vi "Initialize Protection Frames.vi"(8 "error in (no error)":errorcluster, 10 "Frames":T1[](array[typedef]) {"Protection Configurations"."CRC Channels"."Data Type" items=["Signed", "Unsigned", "IEEE Float"]}, 11 "PCL (usec)":u32) -> (0 "error out":errorcluster, 2 "RT Frames":T8[](array[typedef]) {"Protection Configurations"."CRC Channels"."Data Type" items=["Signed", "Unsigned", "IEEE Float"]})   [LabVIEW 2015, in "Protection and Counter Support Engine.lvlib"]
uses:
  Protection and Counter Support Engine.lvlib
  Types/RT Frame Settings.ctl
  Shared/Types/Exported Frame Type.ctl
  Types/RT Protection Configuration.ctl
  Shared/Types/Protection Type.ctl
  Shared/Types/XNET Signal Configuration.ctl
  Shared/Types/Exported Counter Settings.ctl
  Shared/Types/Exported Event Trigger Type.ctl
  Shared/Types/Exported Frame Settings.ctl
  Shared/Types/Exported Protection Settings.ctl
  <vilib>/xnet/xnet.llb/XNET Create Session (Conversion).vi
  Shared/Protection and Counter Support Shared.lvlib
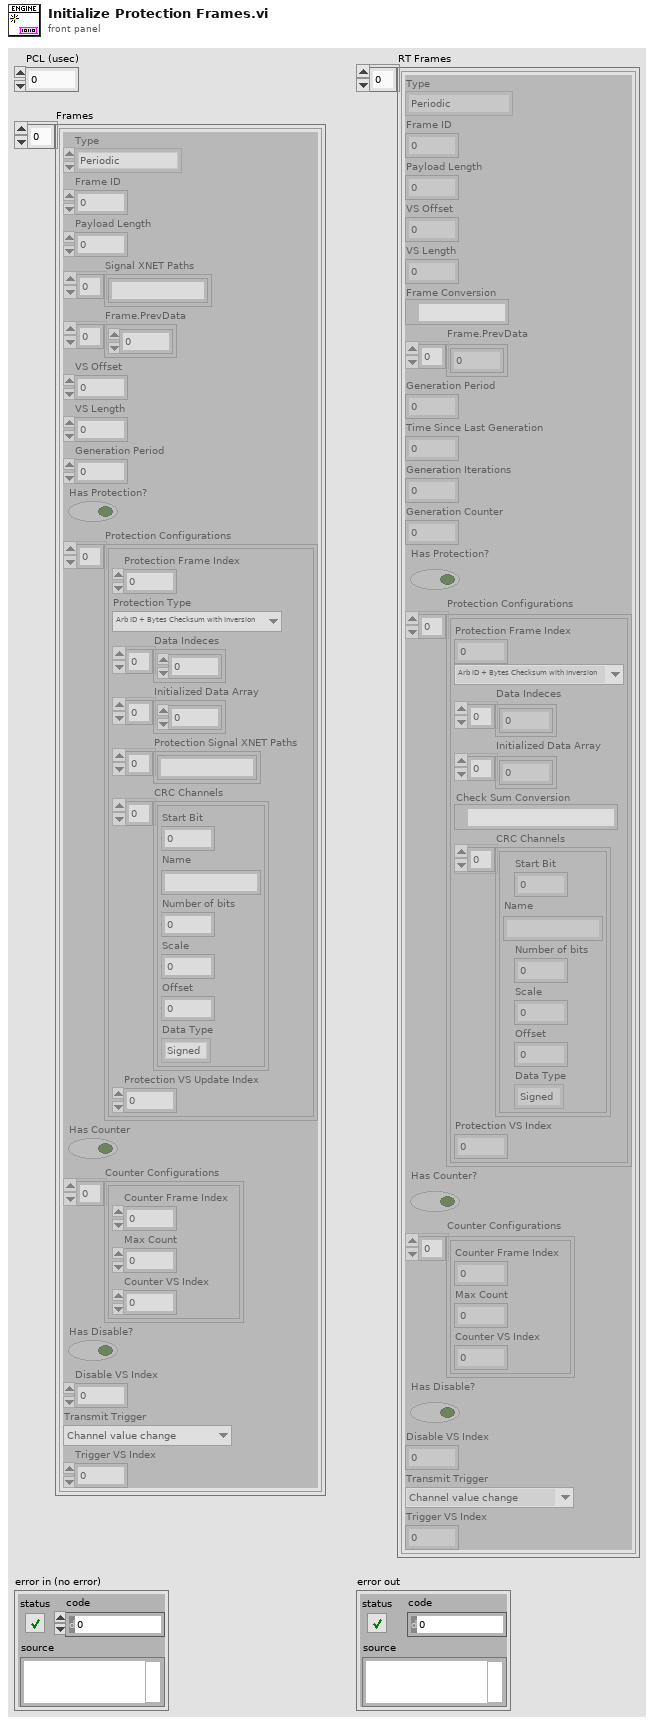
[diagram p1: front panel]
types:
  T1 = typedef "Protection and Counter Support Shared.lvlib/Exported Frame Settings.ctl" = cluster{"Type":T2, "Frame ID":u32, "Payload Length":u32, "Signal XNET Paths":string[], "Frame.PrevData":dbl[], "VS Offset":i32, "VS Length":i32, "Generation Period":u32, "Has Protection?":bool, "Protection Configurations":T3[], "Has Counter":bool, "Counter Configurations":T6[], "Has Disable?":bool, "Disable VS Index":i32, "Transmit Trigger":T7, "Trigger VS Index":i32}
  T2 = typedef "Protection and Counter Support Shared.lvlib/Exported Frame Type.ctl" = enum16{"Periodic", "Event", "Periodic/Event"}
  T3 = typedef "Protection and Counter Support Shared.lvlib/Exported Protection Settings.ctl" = cluster{"Protection Frame Index":i32, "Protection Type":T4, "Data Indeces":i32[], "Initialized Data Array":dbl[], "Protection Signal XNET Paths":string[], "CRC Channels":T5[], "Protection VS Update Index":i32}
  T4 = typedef "Protection and Counter Support Shared.lvlib/Protection Type.ctl" = enum16{"Arb ID + Bytes Checksum with Inversion", "Arb ID + Bytes CRC with Inversion", "Reversed Raw Signal Checksum with Inversion"}
  T5 = typedef "Protection and Counter Support Shared.lvlib/XNET Signal Configuration.ctl" = cluster{"Start Bit":i32, "Name":string, "Number of bits":i32, "Scale":dbl, "Offset":dbl, "Data Type":u32}
  T6 = typedef "Protection and Counter Support Shared.lvlib/Exported Counter Settings.ctl" = cluster{"Counter Frame Index":i32, "Max Count":dbl, "Counter VS Index":i32}
  T7 = typedef "Protection and Counter Support Shared.lvlib/Exported Event Trigger Type.ctl" = enum16{"Channel value change", "Trigger channel (not zero)", "Channel value change or trigger channel (not zero)", "Trigger channel (any value change)", "Channel value change or trigger channel (any value change)"}
  T8 = typedef "Protection and Counter Support Engine.lvlib/RT Frame Settings.ctl" = cluster{"Type":T2, "Frame ID":u32, "Payload Length":u32, "VS Offset":i32, "VS Length":i32, "Frame Conversion":refnum<k21>, "Frame.PrevData":dbl[], "Generation Period":u32, "Time Since Last Generation":u32, "Generation Iterations":u32, "Generation Counter":u32, "Has Protection?":bool, "Protection Configurations":T9[], "Has Counter?":bool, "Counter Configurations":T6[], "Has Disable?":bool, "Disable VS Index":i32, "Transmit Trigger":T7, "Trigger VS Index":i32}
  T9 = typedef "Protection and Counter Support Engine.lvlib/RT Protection Configuration.ctl" = cluster{"Protection Frame Index":i32, "Protection Type":T4, "Data Indeces":i32[], "Initialized Data Array":dbl[], "Check Sum Conversion":refnum<k21>, "CRC Channels":T5[], "Protection VS Index":i32}
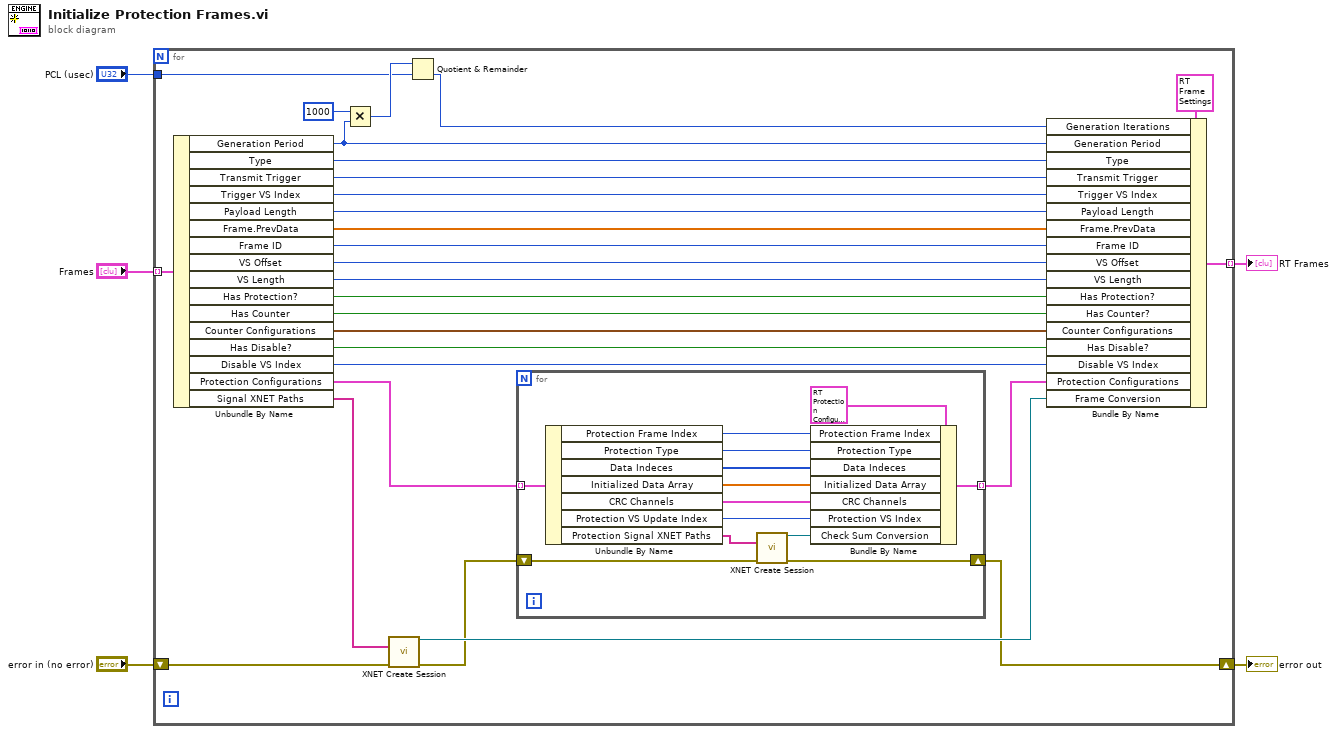
[diagram p0: block diagram]
diagram:
  n1 = for {
    shift-right: [w18] -> w2
    shift-left: "error in (no error)" -> [w31]
    tunnel: "Frames" -> [w33] mode=indexing
    tunnel: [w17] -> w5 mode=indexing
    tunnel: "PCL (usec)" -> [w12]
    n2 = Unbundle By Name(w33) -> ("Generation Period"=w11:u32, "Type"=w6:T2, "Transmit Trigger"=w7:T7, "Trigger VS Index"=w8:i32, "Payload Length"=w9:u32, "Frame.PrevData"=w15:dbl[], "Frame ID"=w29:u32, "VS Offset"=w28:i32, "VS Length"=w27:i32, "Has Protection?"=w26:bool, "Has Counter"=w25:bool, "Counter Configurations"=w24:T6[], "Has Disable?"=w23:bool, "Disable VS Index"=w22:i32, "Protection Configurations"=w21:T3[], "Signal XNET Paths"=w32:string[])
    n3 = Multiply(x=u32 1000, y=w11) -> (x*y=w13:u32)
    n4 = call-poly <vilib>:"XNET Create Session.vi"("signal list"=w32, "error in (no error)"=w31) -> ("session out"=w30:refnum<k21>, "error out"=w19:errorcluster)  [unwired: 12 out]
    n5 = Quotient & Remainder(x=w13, y=w12) -> (floor(x/y)=w10:u32)  [unwired: 1 out]
    n6 = for {
      tunnel: w21 -> [w46] mode=indexing
      tunnel: [w36] -> w20 mode=indexing
      shift-right: [w34] -> w18
      shift-left: w19 -> [w35]
      n7 = Unbundle By Name(w46) -> ("Protection Frame Index"=w44:i32, "Protection Type"=w43:T4, "Data Indeces"=w42:i32[], "Initialized Data Array"=w41:dbl[], "CRC Channels"=w40:T5[], "Protection VS Update Index"=w39:i32, "Protection Signal XNET Paths"=w38:string[])
      n8 = call-poly <vilib>:"XNET Create Session.vi"("signal list"=w38, "error in (no error)"=w35) -> ("session out"=w37:refnum<k21>, "error out"=w34:errorcluster)  [unwired: 12 out]
      n9 = Bundle By Name(cluster=T9 {"Protection Frame Index"=0, "Protection Type"=enum."Arb ID + Bytes Checksum with Inversion", "Data Indeces"=[], "Initialized Data Array"=[], "Check Sum Conversion"="", "CRC Channels"=[], "Protection VS Index"=0} ("Cluster"), "Protection Frame Index"=w44, "Protection Type"=w43, "Data Indeces"=w42, "Initialized Data Array"=w41, "CRC Channels"=w40, "Protection VS Index"=w39, "Check Sum Conversion"=w37) -> (w36:T9)
    }
    n10 = Bundle By Name(cluster=T8 {"Type"=enum."Periodic", "Frame ID"=0, "Payload Length"=0, "VS Offset"=0, "VS Length"=0, "Frame Conversion"="", "Frame.PrevData"=[], "Generation Period"=0, "Time Since Last Generation"=0, "Generation Iterations"=0, "Generation Counter"=0, "Has Protection?"=FALSE, "Protection Configurations"=[], "Has Counter?"=FALSE, "Counter Configurations"=[], "Has Disable?"=FALSE, "Disable VS Index"=0, "Transmit Trigger"=enum."Channel value change", "Trigger VS Index"=0} ("Frame Settings"), "Generation Iterations"=w10, "Generation Period"=w11, "Type"=w6, "Transmit Trigger"=w7, "Trigger VS Index"=w8, "Payload Length"=w9, "Frame.PrevData"=w15, "Frame ID"=w29, "VS Offset"=w28, "VS Length"=w27, "Has Protection?"=w26, "Has Counter?"=w25, "Counter Configurations"=w24, "Has Disable?"=w23, "Disable VS Index"=w22, "Protection Configurations"=w20, "Frame Conversion"=w30) -> (w17:T8)
  }
  "RT Frames" <- w5
  "error out" <- w2
